vi "Fetch.vi"(8 "error in (no error)":errorcluster, 11 "HP3458aDMM in":refnum<class "HP3458aDMM.lvclass">) -> (0 "error out":errorcluster, 3 "HP3458aDMM out":refnum<class "HP3458aDMM.lvclass">)   [LabVIEW 2014, in "SamplerPlugins.lvlib" / "HP3458aDMM.lvclass"]
uses:
  HP3458aDMM.lvclass
  <instrlib>/Agilent 3458/Agilent 3458.lvlib
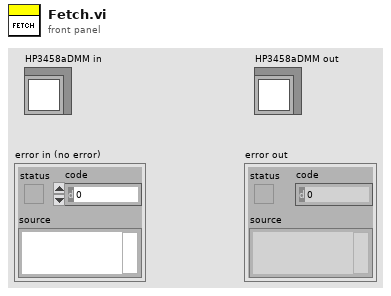
[diagram p1: front panel]
types:
  T1 = enum16{"ASCII", "Single Real", "Double Real", "Single Integer", "Double Integer"}
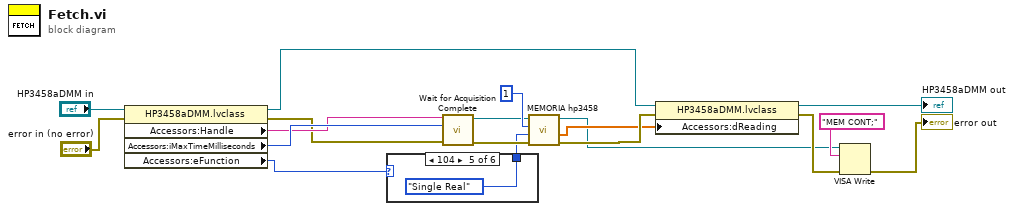
[diagram p0: block diagram]
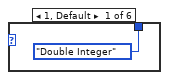
[diagram p2: hidden frame]
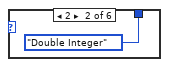
[diagram p3: hidden frame]
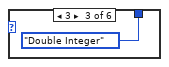
[diagram p4: hidden frame]
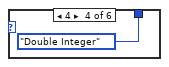
[diagram p5: hidden frame]
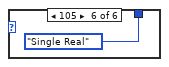
[diagram p6: hidden frame]
diagram:
  n1 = property class="HP3458aDMM.lvclass"(reference="HP3458aDMM in", error in="error in (no error)") -> (reference out=w18:refnum<class "HP3458aDMM.lvclass">, error out=w11:errorcluster, "Accessors:Handle"=w12:string, "Accessors:iMaxTimeMilliseconds"=w14:i32, "Accessors:eFunction"=w9:u16)
  n2 = case shown="104" w9 {
    tunnel: [T1."Double Integer" ("Output Format (0:ASCII)") T1."Double Integer" ("Output Format (0:ASCII)") T1."Double Integer" ("Output Format (0:ASCII)") T1."Double Integer" ("Output Format (0:ASCII)") T1."Single Real" ("Output Format (0:ASCII)") T1."Single Real" ("Output Format (0:ASCII)")] -> w3
    frame 1, Default {
    }
    frame 2 {
    }
    frame 3 {
    }
    frame 4 {
    }
    frame 104 {
    }
    frame 105 {
    }
  }
  n3 = call <instrlib>:"Wait for Acquisition Complete.vi"("error in (no error)"=w11, "Maximum Time (10000 ms)"=w14, "VISA resource name"=w12) -> ("error out"=w4:errorcluster, "VISA resource name out"=w1:refnum<visa-resource-name>)  [unwired: 7 in]
  n4 = call "MEMORIA hp3458.vi"("error in (no error)"=w4, "Output Format (0:ASCII)"=w3, "Número de muestras totales"=1, "VISA session"=w1) -> ("error out"=w13:errorcluster, "Muestras digitales"=w10:dbl[], "dup VISA session"=w5:refnum<visa-resource-name>)  [unwired: 4 in, 1 out]
  n5 = property class="HP3458aDMM.lvclass"(reference=w18, error in=w13, "Accessors:dReading"=w10) -> (reference out=→"HP3458aDMM out":refnum<class "HP3458aDMM.lvclass">, error out=w7:errorcluster)
  n6 = VISA Write(VISA resource name=w5, write buffer="MEM CONT;", error in (no error)=w7) -> (error out=→"error out":errorcluster)  [unwired: 2 out]
